vi "getFPGA.vi"(11 "Model in":refnum<class "Model.lvclass">) -> (2 "FPGA":refnum<class "FPGA.lvclass">, 3 "Model out":refnum<class "Model.lvclass">)   [LabVIEW 2016, in "Model.lvclass"]
uses:
  Model.lvclass
  Resources/FPGA/FPGA.lvclass
  Model.lvclass/Model.ctl
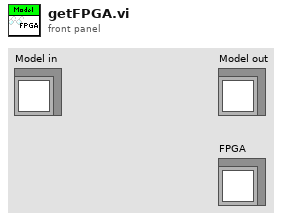
[diagram p1: front panel]
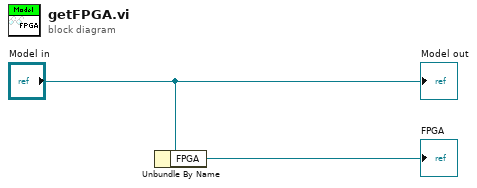
[diagram p0: block diagram]
diagram:
  n1 = Unbundle By Name("Model in") -> ("FPGA"=→"FPGA":refnum<class "FPGA.lvclass">)
  "Model out" <- "Model in"
